vi "Abort Trial.vi"(8 "error in (no error)":errorcluster, 9 "Input Params":cluster{"Name":string, "Data":variant}[](array[cluster]), 10 "Abort Reason":string, 11 "Matlab Connection":refnum<k5>) -> (0 "error out":errorcluster, 1 "Return value struct":cluster{"Name":string, "Data":variant}[](array[cluster]), 2 "Return value I32":i32, 3 "connection ID out":refnum<k5>)   [LabVIEW 2010, in "Matlab API.lvlib"]
uses:
  Matlab API.lvlib
  Core SubVIs/Core SubVIs.lvlib
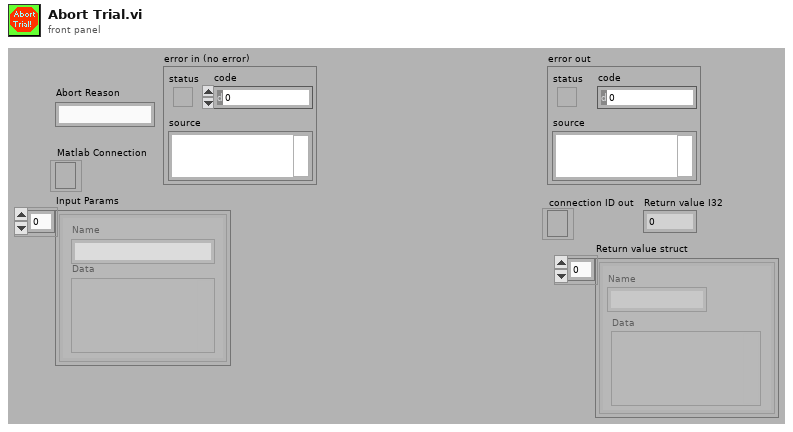
[diagram p1: front panel]
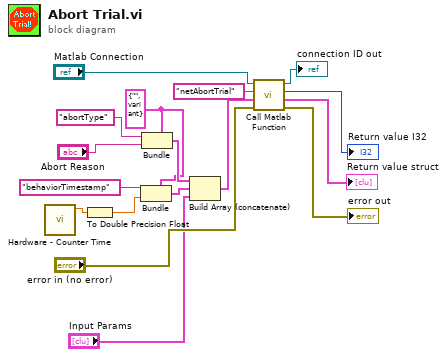
[diagram p0: block diagram]
diagram:
  w4 = cluster{"Name":string, "Data":variant} {"Name"="", "Data"=variant} ("Cluster")
  n1 = call "Hardware - Counter Time.vi"() -> ("Timer Value (ms)"=w16:dbl)  [unwired: 3 in, 8 out]
  n2 = To Double Precision Float(number=w16) -> (double precision float=w7:dbl)
  n3 = Bundle(cluster=w4, "Name"="behaviorTimestamp" ("Variable name"), "Data"=w7) -> (w6:cluster{"Name":string, "Data":variant})
  n4 = Bundle(cluster=w4, "Name"="abortType" ("Variable name"), "Data"="Abort Reason") -> (w9:cluster{"Name":string, "Data":variant})
  n5 = Build Array (concatenate)(w9, w6, "Input Params") -> (w15:cluster{"Name":string, "Data":variant}[])
  n6 = call "Call Matlab Function.vi"("error in (no error)"="error in (no error)", "Matlab Param Array"=w15, "Function name"="netAbortTrial", "TCP Network Connection Refnum"="Matlab Connection") -> ("error out"=→"error out":errorcluster, "Return value struct"=→"Return value struct":cluster{"Name":string, "Data":variant}[], "Return value I32"=→"Return value I32":i32, "connection ID out"=→"connection ID out":refnum<k5>)  [unwired: 4 out]
